vi "PicoReadPicoStreamingBuffers.vi"(1 "enabled array":i16[](array[numeric]), 2 "Buffer and Transfer Settings":T2={"startIndex"=0, "Samples"=1000000, "Down Sample Ratio"=1, "Down-Sample Mode"=2147483648} {"Down-Sample Mode" items=["None"=2147483648, "Aggregate"=1, "Decimate"=2, "Average"=4]; "Down Sample Ratio" step=1; "Samples" format="%_6p"}, 3 "Variant":string, 5 "Pointer array":u64[][](array[numeric]), 7 "Offset Index":u32, 9 "Number of Samples":u32, 11 "error in (no error)":errorcluster) -> (6 "Buffers (Max or non-aggregated)":T1, 8 "Buffers (Min)":T1, 15 "error out":errorcluster)   [LabVIEW 2010]
doc: "Read data from Picodata buffers for streaming examples"
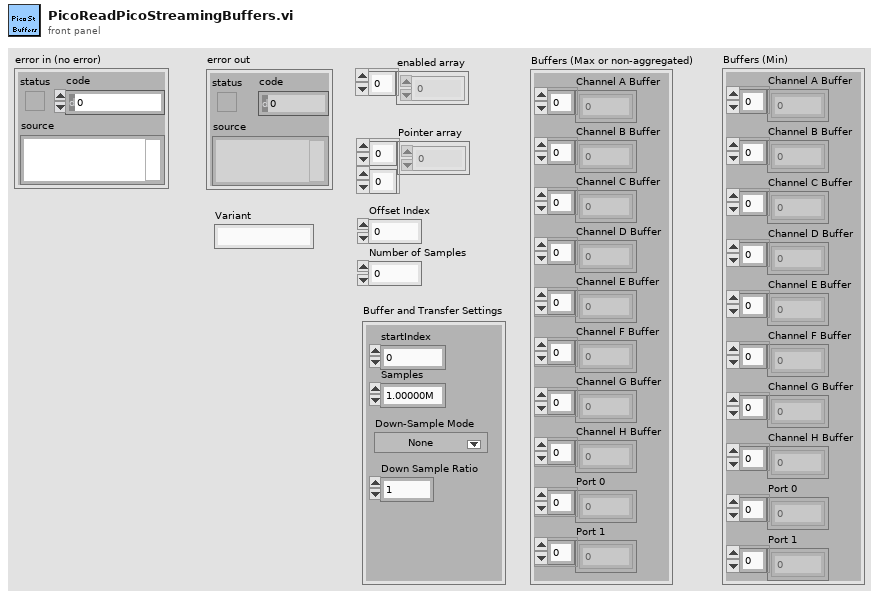
[diagram p1: front panel]
types:
  T1 = cluster{"Channel A Buffer":i16[], "Channel B Buffer":i16[], "Channel C Buffer":i16[], "Channel D Buffer":i16[], "Channel E Buffer":i16[], "Channel F Buffer":i16[], "Channel G Buffer":i16[], "Channel H Buffer":i16[], "Port 0":i16[], "Port 1":i16[]}
  T2 = cluster{"startIndex":u64, "Samples":u64, "Down Sample Ratio":u64, "Down-Sample Mode":u32}
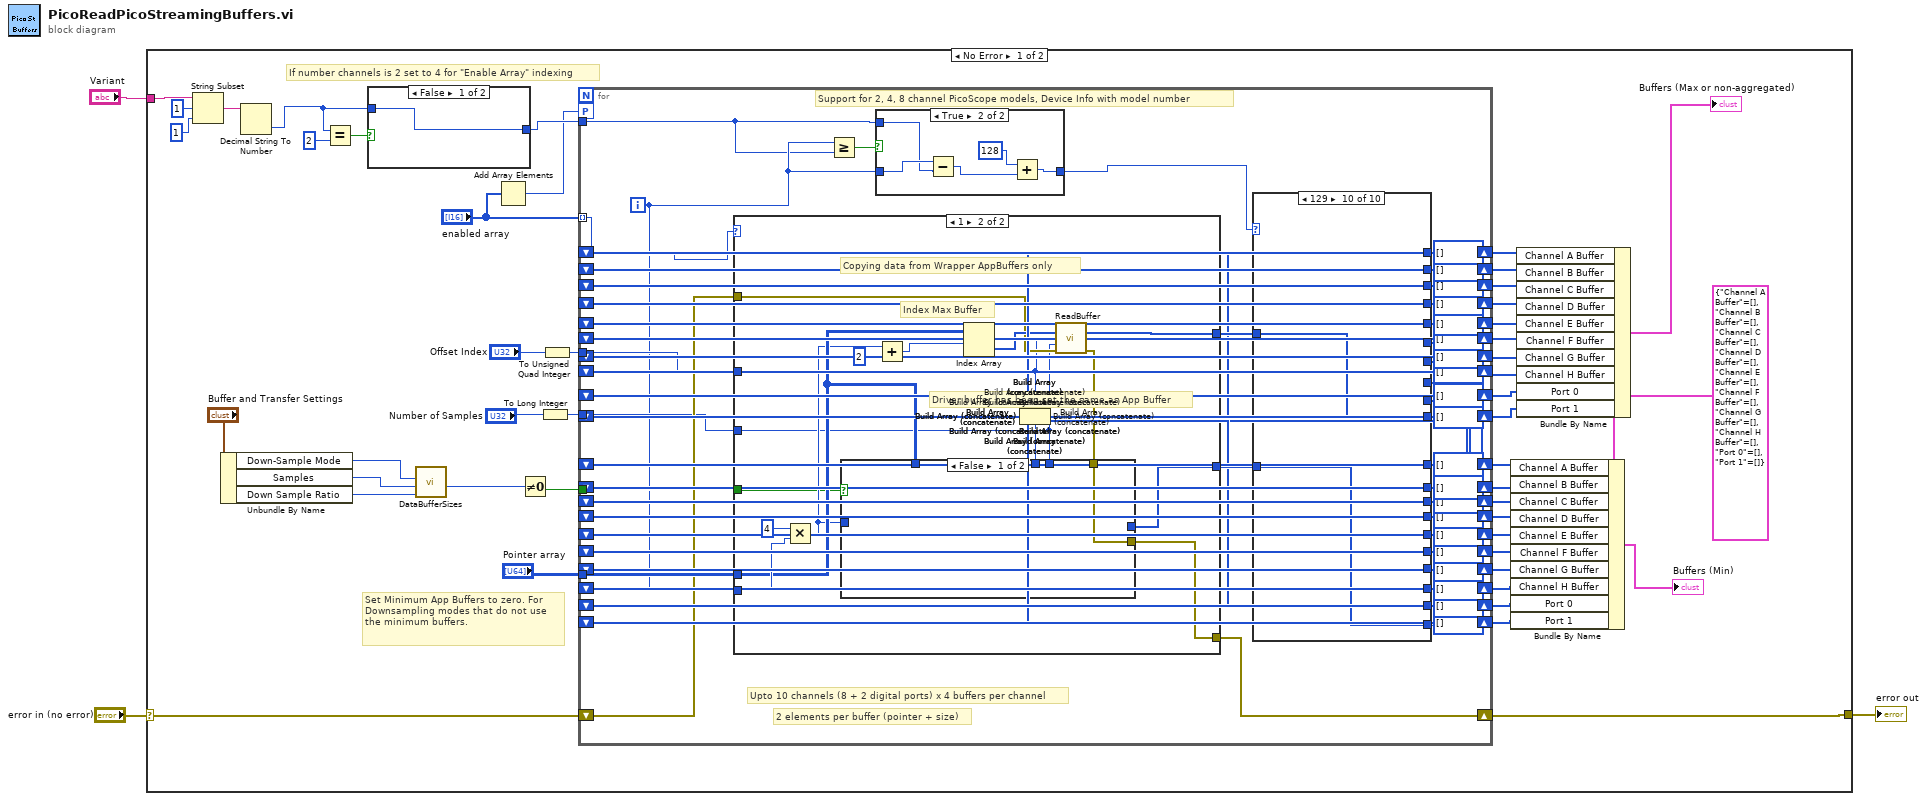
[diagram p0: block diagram]
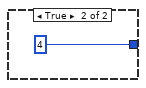
[diagram p2: hidden frame]
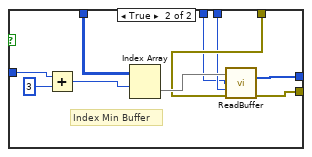
[diagram p14: hidden frame]
diagram:
  n1 = case shown="No Error" "error in (no error)" {
    selector: "error in (no error)" -> [w66 w198]
    tunnel: [w68 w198] -> w2
    tunnel: "Variant" -> [w30 _]
    frame No Error {
      w43 = T1 {"Channel A Buffer"=[], "Channel B Buffer"=[], "Channel C Buffer"=[], "Channel D Buffer"=[], "Channel E Buffer"=[], "Channel F Buffer"=[], "Channel G Buffer"=[], "Channel H Buffer"=[], "Port 0"=[], "Port 1"=[]} ("Buffers (Max or non-aggregated)")
      # "If number channels is 2 set to 4 for \"Enable Array\" indexing"
      # "Set Minimum App Buffers to zero. For Downsampling modes that do not use the minimum buffers."
      n2 = String Subset(string=w30, offset (0)=1, length (rest)=1 ("length (rest)")) -> (substring=w27:string)
      n3 = Unbundle By Name("Buffer and Transfer Settings") -> ("Down-Sample Mode"=w53:u32, "Samples"=w52:u64, "Down Sample Ratio"=w54:u64)
      n4 = Decimal String To Number(string=w27) -> (number=w26:i32)  [unwired: 2 in, 1 out]
      n5 = Equal?(x=w26, y=2 ("Number of channels")) -> (x = y?=w33:bool)
      n6 = case shown="False" w33 {
        tunnel: [w70 4 ("Number of channels")] -> w32
        tunnel: w26 -> [w70 _]
        frame False {
        }
        frame True {
        }
      }
      n7 = call "DataBufferSizes.vi"("Down Sample Ratio"=w54, "Number of Samples"=w52, "Down-Sample Mode"=w53) -> ("min Buffer Size"=w50:i32)  [unwired: 7 in, 1 out]
      n8 = Add Array Elements(numeric array="enabled array") -> (sum=w24:i16)
      n9 = Not Equal To 0?(x=w50) -> (x != 0?=w51:bool)
      n10 = To Long Integer(number="Number of Samples") -> (32bit integer=w45:i32)
      n11 = To Unsigned Quad Integer(1:"Offset Index") -> (0:w48:u64)
      n12 = for {
        tunnel: "enabled array" -> [w143] mode=indexing
        tunnel: "Pointer array" -> [w144]
        shift-right: [w142] -> w68
        shift-left: w66 -> [w141]
        tunnel: w45 -> [w127]
        tunnel: w51 -> [w126]
        tunnel: w48 -> [w124]
        tunnel: w32 -> [w112]
        workers-P: w24 -> [_]
        shift-right: [w110] -> w65
        shift-left: i16[] [] ("Output Array") -> [w111]
        shift-right: [w108] -> w64
        shift-left: i16[] [] ("Output Array") -> [w109]
        shift-right: [w106] -> w63
        shift-left: i16[] [] ("Output Array") -> [w107]
        shift-right: [w104] -> w62
        shift-left: i16[] [] ("Output Array") -> [w105]
        shift-right: [w102] -> w61
        shift-left: i16[] [] ("Output Array") -> [w103]
        shift-right: [w100] -> w60
        shift-left: i16[] [] ("Output Array") -> [w101]
        shift-right: [w98] -> w49
        shift-left: i16[] [] ("Output Array") -> [w99]
        shift-right: [w96] -> w59
        shift-left: i16[] [] ("Output Array") -> [w97]
        shift-right: [w94] -> w58
        shift-left: i16[] [] ("Output Array") -> [w95]
        shift-right: [w92] -> w57
        shift-left: i16[] [] ("Output Array") -> [w93]
        shift-right: [w90] -> w56
        shift-left: i16[] [] ("Output Array") -> [w91]
        shift-right: [w88] -> w55
        shift-left: i16[] [] ("Output Array") -> [w89]
        shift-right: [w86] -> w40
        shift-left: i16[] [] ("Output Array") -> [w87]
        shift-right: [w84] -> w39
        shift-left: i16[] [] ("Output Array") -> [w85]
        shift-right: [w82] -> w41
        shift-left: i16[] [] ("Output Array") -> [w83]
        shift-right: [w80] -> w38
        shift-left: i16[] [] ("Output Array") -> [w81]
        shift-right: [w78] -> w37
        shift-left: i16[] [] ("Output Array") -> [w79]
        shift-right: [w76] -> w36
        shift-left: i16[] [] ("Output Array") -> [w77]
        shift-right: [w74] -> w35
        shift-left: i16[] [] ("Output Array") -> [w75]
        shift-right: [w72] -> w34
        shift-left: i16[] [] ("Output Array") -> [w73]
        i -> [w114]
        # "Support for 2, 4, 8 channel PicoScope models, Device Info with model number"
        # "2 elements per buffer (pointer + size)"
        # "Upto 10 channels (8 + 2 digital ports) x 4 buffers per channel"
        n13 = case shown="1" w143 {
          tunnel: w144 -> [_ w184]
          tunnel: w114 -> [_ w185]
          tunnel: [_ w179] -> w140
          tunnel: [_ w178] -> w139
          tunnel: w141 -> [w171 w177]
          tunnel: [w171 w175] -> w142
          tunnel: w127 -> [_ w173]
          tunnel: w126 -> [_ w174]
          tunnel: w124 -> [_ w172]
          frame 0, Default {
          }
          frame 1 {
            # "Driver buffer has been set the same as App Buffer"
            # "Copying data from Wrapper AppBuffers only"
            # "Index Max Buffer"
            n14 = Multiply(x=4, y=w185) -> (x*y=w181:i32)
            n15 = Add(x=w181, y=2) -> (x+y=w183:i32)
            n16 = Index Array(array=w184, index (row)=w183) -> (element=w180:u64[])  [unwired: 1 in]
            n17 = call "ReadBuffer.vi"("Pointer and BufferSize"=w180, "Offset"=w172, "Buffer size"=w173, "error in (no error)"=w177) -> ("Output Array"=w179:i16[], "error out"=w176:errorcluster)  [unwired: 10 in]
            n18 = case shown="False" w174 {
              tunnel: w184 -> [_ w197]
              tunnel: w181 -> [_ w194]
              tunnel: [_ w192] -> w178
              tunnel: w176 -> [w187 w191]
              tunnel: [w187 w190] -> w175
              tunnel: w173 -> [_ w189]
              tunnel: w172 -> [_ w188]
              frame False {
              }
              frame True {
                # "Index Min Buffer"
                n19 = Add(x=w194, y=3) -> (x+y=w195:i32)
                n20 = Index Array(array=w197, index (row)=w195) -> (element=w193:u64[])  [unwired: 1 in]
                n21 = call "ReadBuffer.vi"("Pointer and BufferSize"=w193, "Offset"=w188, "Buffer size"=w189, "error in (no error)"=w191) -> ("Output Array"=w192:i16[], "error out"=w190:errorcluster)  [unwired: 10 in]
              }
            }
          }
        }
        n22 = Greater Or Equal?(x=w114, y=w112) -> (x >= y?=w115:bool)
        n23 = case shown="True" w115 {
          tunnel: w114 -> [w145 w147]
          tunnel: [w145 w149] -> w113
          tunnel: w112 -> [_ w146]
          frame False {
          }
          frame True {
            n24 = Subtract(x=w147, y=w146) -> (x-y=w148:i32)
            n25 = Add(x=128, y=w148) -> (x+y=w149:i32)
          }
        }
        n26 = case shown="129" w113 {
          tunnel: w140 -> [w152 w154 w156 w158 w160 w162 w164 w166 w168 w169]
          tunnel: [w152 _ _ _ _ _ _ _ _ _] -> w125
          tunnel: [_ w154 _ _ _ _ _ _ _ _] -> w132
          tunnel: [_ _ w156 _ _ _ _ _ _ _] -> w131
          tunnel: [_ _ _ w158 _ _ _ _ _ _] -> w130
          tunnel: [_ _ _ _ w160 _ _ _ _ _] -> w129
          tunnel: [_ _ _ _ _ w162 _ _ _ _] -> w128
          tunnel: w139 -> [w151 w153 w155 w157 w159 w161 w163 w165 w167 w170]
          tunnel: [w151 _ _ _ _ _ _ _ _ _] -> w138
          tunnel: [_ w153 _ _ _ _ _ _ _ _] -> w137
          tunnel: [_ _ w155 _ _ _ _ _ _ _] -> w136
          tunnel: [_ _ _ w157 _ _ _ _ _ _] -> w135
          tunnel: [_ _ _ _ w159 _ _ _ _ _] -> w134
          tunnel: [_ _ _ _ _ w161 _ _ _ _] -> w133
          tunnel: [_ _ _ _ _ _ w164 _ _ _] -> w123
          tunnel: [_ _ _ _ _ _ _ w166 _ _] -> w122
          tunnel: [_ _ _ _ _ _ w163 _ _ _] -> w121
          tunnel: [_ _ _ _ _ _ _ w165 _ _] -> w120
          tunnel: [_ _ _ _ _ _ _ _ w168 _] -> w119
          tunnel: [_ _ _ _ _ _ _ _ w167 _] -> w118
          tunnel: [_ _ _ _ _ _ _ _ _ w170] -> w117
          tunnel: [_ _ _ _ _ _ _ _ _ w169] -> w116
          frame 0, Default {
          }
          frame 1 {
          }
          frame 2 {
          }
          frame 3 {
          }
          frame 4 {
          }
          frame 5 {
          }
          frame 6 {
          }
          frame 7 {
          }
          frame 128 {
          }
          frame 129 {
          }
        }
        n27 = Build Array (concatenate)(w73, w116) -> (w72:i16[])
        n28 = Build Array (concatenate)(w75, w117) -> (w74:i16[])
        n29 = Build Array (concatenate)(w77, w118) -> (w76:i16[])
        n30 = Build Array (concatenate)(w79, w119) -> (w78:i16[])
        n31 = Build Array (concatenate)(w81, w120) -> (w80:i16[])
        n32 = Build Array (concatenate)(w83, w121) -> (w82:i16[])
        n33 = Build Array (concatenate)(w85, w122) -> (w84:i16[])
        n34 = Build Array (concatenate)(w87, w123) -> (w86:i16[])
        n35 = Build Array (concatenate)(w89, w128) -> (w88:i16[])
        n36 = Build Array (concatenate)(w91, w129) -> (w90:i16[])
        n37 = Build Array (concatenate)(w93, w130) -> (w92:i16[])
        n38 = Build Array (concatenate)(w95, w131) -> (w94:i16[])
        n39 = Build Array (concatenate)(w97, w132) -> (w96:i16[])
        n40 = Build Array (concatenate)(w99, w125) -> (w98:i16[])
        n41 = Build Array (concatenate)(w101, w133) -> (w100:i16[])
        n42 = Build Array (concatenate)(w103, w134) -> (w102:i16[])
        n43 = Build Array (concatenate)(w105, w135) -> (w104:i16[])
        n44 = Build Array (concatenate)(w107, w136) -> (w106:i16[])
        n45 = Build Array (concatenate)(w109, w137) -> (w108:i16[])
        n46 = Build Array (concatenate)(w111, w138) -> (w110:i16[])
      }
      n47 = Bundle By Name(cluster=w43, "Channel A Buffer"=w65, "Channel B Buffer"=w64, "Channel C Buffer"=w63, "Channel D Buffer"=w62, "Channel E Buffer"=w61, "Channel F Buffer"=w60, "Channel G Buffer"=w41, "Channel H Buffer"=w38, "Port 0"=w36, "Port 1"=w35) -> (→"Buffers (Min)":T1)
      n48 = Bundle By Name(cluster=w43, "Channel A Buffer"=w49, "Channel B Buffer"=w59, "Channel C Buffer"=w58, "Channel D Buffer"=w57, "Channel E Buffer"=w56, "Channel F Buffer"=w55, "Channel G Buffer"=w40, "Channel H Buffer"=w39, "Port 0"=w37, "Port 1"=w34) -> (→"Buffers (Max or non-aggregated)":T1)
    }
    frame Error {
    }
  }
  "error out" <- w2
